vi "CRYNotch Resonance Results.vi"(9 "Y ref":dbl=1.0, 10 "Input":cluster{"Freq":dbl, "Magn":dbl}[](array[cluster]) {"Magn" format="%.4f"; "Freq" format="%.2f"}, 11 "Y data":dbl=1.0) -> (0 "Output":cluster{"FStart":dbl, "Magn":dbl}[](array[cluster]) {"Magn" format="%.2f"; "FStart" format="%.2f"}, 1 "Q":dbl format="%.2f", 2 "Magn":dbl format="%.2f", 3 "Freq":dbl format="%.2f")   [LabVIEW 2013]
uses:
  <vilib>/Analysis/7linalg.llb/Solve Linear Equations (single right hand).vi
  <vilib>/Analysis/baseanly.llb/Solve Linear Equations By Cholesky.vi
  <vilib>/Analysis/baseanly.llb/Real Matrix to Compact Array.vi
  <vilib>/Analysis/baseanly.llb/Real Compact Tri-Matrix Linear Eqs.vi
  <vilib>/Analysis/NI_AALPro.lvlib
panel:
  out "error":i32
  in  "Algorithm (0)":i32 min=0 max=2 step=1
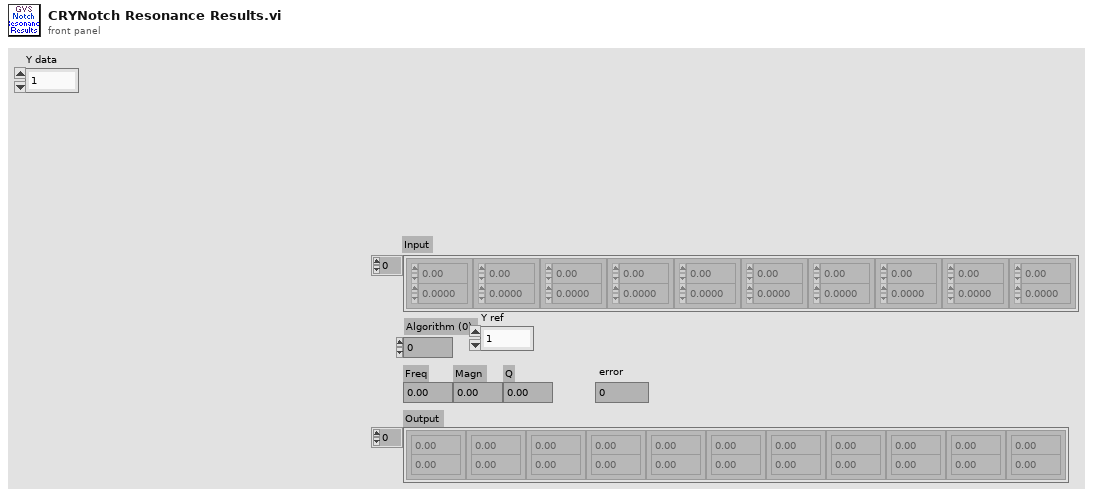
[diagram p1: front panel]
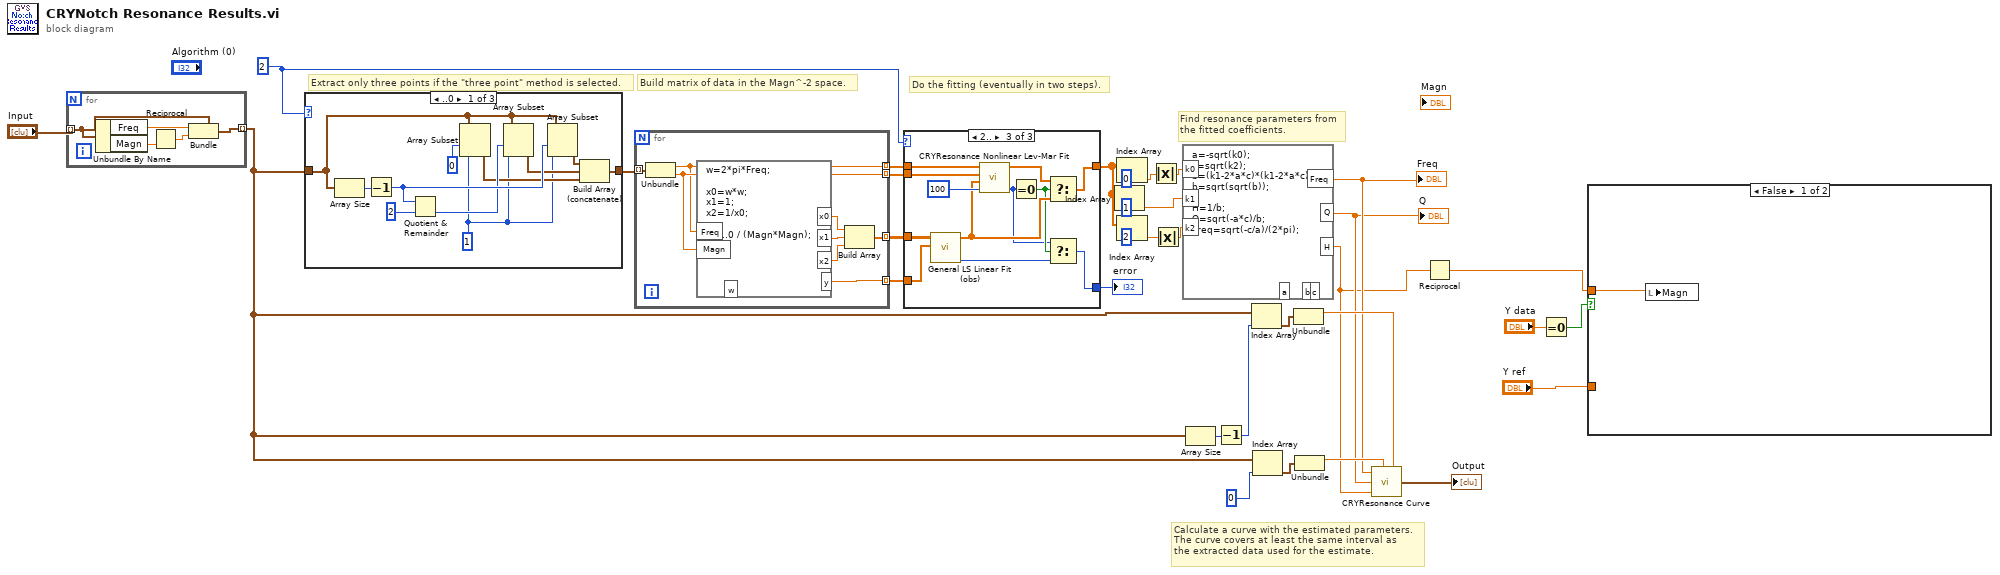
[diagram p0: block diagram]
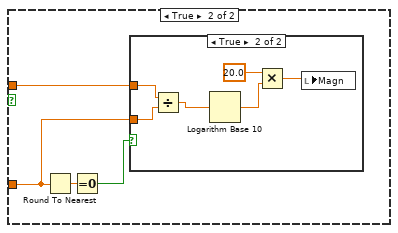
[diagram p2: hidden frame]
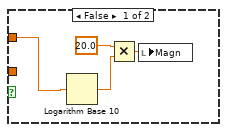
[diagram p3: hidden frame]
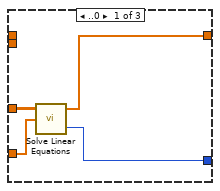
[diagram p4: hidden frame]
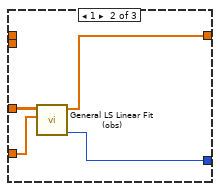
[diagram p5: hidden frame]
diagram:
  w14 = 2
  # "Calculate a curve with the estimated parameters. \nThe curve covers at least the same interval as\nthe extracted data used for the estimate."
  # "Find resonance parameters from\nthe fitted coefficients."
  # "Do the fitting (eventually in two steps)."
  # "Build matrix of data in the Magn^-2 space."
  # "Extract only three points if the \"three point\" method is selected."
  n1 = for {
    tunnel: "Input" -> [w36] mode=indexing
    tunnel: [w37] -> w4 mode=indexing
    n2 = Unbundle By Name(w36) -> ("Freq"=w38:dbl, "Magn"=w35:dbl)
    n3 = Reciprocal(x=w35) -> (1/x=w34:dbl)
    n4 = Bundle(cluster=w36, "Freq"=w38, "Magn"=w34) -> (w37:cluster{"Freq":dbl, "Magn":dbl})
  }
  n5 = case shown="..0" w14 {
    tunnel: w4 -> [w39 w50 w51]
    tunnel: [w40 w50 w51] -> w29
    frame ..0 {
      w41 = 1
      n6 = Array Size(array=w39) -> (size(s)=w48:i32)
      n7 = Decrement(x=w48) -> (x-1=w49:i32)
      n8 = Quotient & Remainder(x=w49, y=2) -> (floor(x/y)=w46:i32)  [unwired: 1 out]
      n9 = Array Subset(array=w39, index=0, length=w41) -> (w45:cluster{"Freq":dbl, "Magn":dbl}[])
      n10 = Array Subset(array=w39, index=w46, length=w41) -> (w44:cluster{"Freq":dbl, "Magn":dbl}[])
      n11 = Array Subset(array=w39, index=w49, length=w41) -> (w43:cluster{"Freq":dbl, "Magn":dbl}[])
      n12 = Build Array (concatenate)(w43, w44, w45) -> (w40:cluster{"Freq":dbl, "Magn":dbl}[])
    }
    frame 1 {
    }
    frame 2.. {
    }
  }
  n13 = for {
    tunnel: w29 -> [w59] mode=indexing
    tunnel: [w56] -> w28 mode=indexing
    tunnel: [w53] -> w27 mode=indexing
    tunnel: [w52] -> w25 mode=indexing
    tunnel: [w58] -> w26 mode=indexing
    n14 = Unbundle(w59) -> ("Freq"=w52:dbl, "Magn"=w58:dbl)
    n15 = formula code="w=2*pi*Freq;\n\nx0=w*w;\nx1=1;\nx2=1/x0;\n\ny=1.0 / (Magn*Magn);"("Freq"=w52, "Magn"=w58) -> ("x0"=w57:dbl, "x1"=w55:dbl, "x2"=w54:dbl, "y"=w53:dbl)  [unwired: 1 out]
    n16 = Build Array(w57, w55, w54) -> (w56:dbl[])
  }
  n17 = case shown="2.." w14 {
    tunnel: w28 -> [w63 w67 w78]
    tunnel: w27 -> [w62 w66 w77]
    tunnel: w26 -> [_ _ w76]
    tunnel: w25 -> [_ _ w75]
    tunnel: [w61 w65 w72] -> w24
    tunnel: [w60 w64 w68] -> w15
    frame ..0 {
      n18 = call-poly <vilib>:"Solve Linear Equations.vi"("Known Vector"=w62, "Input Matrix"=w63) -> ("error"=w60:i32, "Solution Vector"=w61:dbl[])  [unwired: 1 in]
    }
    frame 1 {
      n19 = call <vilib>:"General LS Linear Fit (obs).vi"("H"=w67, "Y"=w66) -> ("Coefficients"=w65:dbl[], "error"=w64:i32)  [unwired: 3 in, 3 out]
    }
    frame 2.. {
      n20 = call <vilib>:"General LS Linear Fit (obs).vi"("H"=w78, "Y"=w77) -> ("Coefficients"=w74:dbl[], "error"=w70:i32)  [unwired: 3 in, 3 out]
      n21 = call "CRYResonance Nonlinear Lev-Mar Fit.vi"("max iteration"=100, "Initial Guess Coefficients"=w74, "Y"=w76, "X"=w75) -> ("error"=w69:i32, "Best Fit Coefficients"=w73:dbl[])  [unwired: 2 in, 3 out]
      n22 = Equal To 0?(x=w69) -> (x = 0?=w71:bool)
      n23 = Select(t=w73, s=w71, f=w74) -> (s? t:f=w72:dbl[])
      n24 = Select(t=w69, s=w71, f=w70) -> (s? t:f=w68:i32)
    }
  }
  "error" <- w15
  n25 = Index Array(array=w24, index=1) -> (element=w30:dbl)
  n26 = Index Array(array=w24, index=0) -> (element=w11:dbl)
  n27 = Index Array(array=w24, index=2) -> (element=w9:dbl)
  n28 = Absolute Value(x=w11) -> (abs(x)=w10:dbl)
  n29 = Absolute Value(x=w9) -> (abs(x)=w8:dbl)
  n30 = formula code="a=-sqrt(k0);\nc=sqrt(k2);\nb=(k1-2*a*c)*(k1-2*a*c);\nb=sqrt(sqrt(b));\n\nH=1/b;\nQ=sqrt(-a*c)/b;\nFreq=sqrt(-c/a)/(2*pi);"("k0"=w10, "k1"=w30, "k2"=w8) -> ("Q"=w12:dbl, "Freq"=w13:dbl, "H"=w1:dbl)  [unwired: 3 out]
  "Freq" <- w13
  "Q" <- w12
  n31 = Array Size(array=w4) -> (size(s)=w22:i32)
  n32 = Decrement(x=w22) -> (x-1=w21:i32)
  n33 = Index Array(array=w4, index=w21) -> (element=w19:cluster{"Freq":dbl, "Magn":dbl})
  n34 = Index Array(array=w4, index=0) -> (element=w18:cluster{"Freq":dbl, "Magn":dbl})
  n35 = Unbundle(w19) -> ("Freq"=w17:dbl)  [unwired: 1 out]
  n36 = Unbundle(w18) -> ("Freq"=w16:dbl)  [unwired: 1 out]
  n37 = call "CRYResonance Curve.vi"("Freq"=w13, "Low Freq"=w16, "Q"=w12, "Magn"=w1, "High Freq"=w17) -> ("Output"=→"Output":cluster{"FStart":dbl, "Magn":dbl}[])  [unwired: 2 in, 2 out]
  n38 = Reciprocal(x=w1) -> (1/x=w2:dbl)
  n39 = Equal To 0?(x="Y data") -> (x = 0?=w5:bool)
  n40 = case shown="False" w5 {
    tunnel: w2 -> [w80 w82]
    tunnel: "Y ref" -> [_ w81]
    frame False {
      n41 = local write "Magn"(w80) -> ()
    }
    frame True {
      n42 = Round To Nearest(number=w81) -> (nearest integer value=w84:dbl)
      n43 = Equal To 0?(x=w84) -> (x = 0?=w83:bool)
      n44 = case shown="True" w83 {
        tunnel: w82 -> [w85 w94]
        tunnel: w81 -> [_ w93]
        frame False {
          n45 = Logarithm Base 10(1:w85) -> (0:w86:dbl)
          n46 = Multiply(x=20.0, y=w86) -> (x*y=w88:dbl)
          n47 = local write "Magn"(w88) -> ()
        }
        frame True {
          n48 = Divide(x=w94, y=w93) -> (x/y=w90:dbl)
          n49 = Logarithm Base 10(1:w90) -> (0:w91:dbl)
          n50 = Multiply(x=20.0, y=w91) -> (x*y=w89:dbl)
          n51 = local write "Magn"(w89) -> ()
        }
      }
    }
  }
